vi "nonlinear spring simulation.vi"(7 "Solver Params":T1={"Initial Time"=0.0, "Final Time"=10.0, "Time Step"=0.1, "Absolute Tolerance"=0.001, "Relative Tolerance"=1e-07, "Solver Method"=enum."Runge-Kutta 4", "Discrete Time Step"=0.1, "Minimum Time Step"=0.01, "Maximum Time Step"=0.1, "Initial Time Step"=0.01} {"Initial Time Step" min=0.0; "Maximum Time Step" min=0.0; "Minimum Time Step" min=0.0; "Discrete Time Step" min=0.0; "Relative Tolerance" min=0.0; "Absolute Tolerance" min=0.0; "Time Step" min=0.0}, 8 "Error In":errorcluster, 9 "xp Noise STD":dbl(knob)=0.05 scale=0.0..0.1, 10 "Spring Constant":dbl(knob)=2.0 scale=0.0..10.0, 11 "Initial Conditions":dbl[](array[numeric])=[1.0, 0.0]) -> (0 "Error Out":errorcluster, 2 "times":dbl[](array[numeric]), 3 "outputs":dbl[][](array[numeric]))   [LabVIEW 2023]
doc: "Nonlinear spring simulation"
uses:
  <vilib>/gmath/NI_Gmath.lvlib
  <vilib>/Analysis/NI_AALBase.lvlib
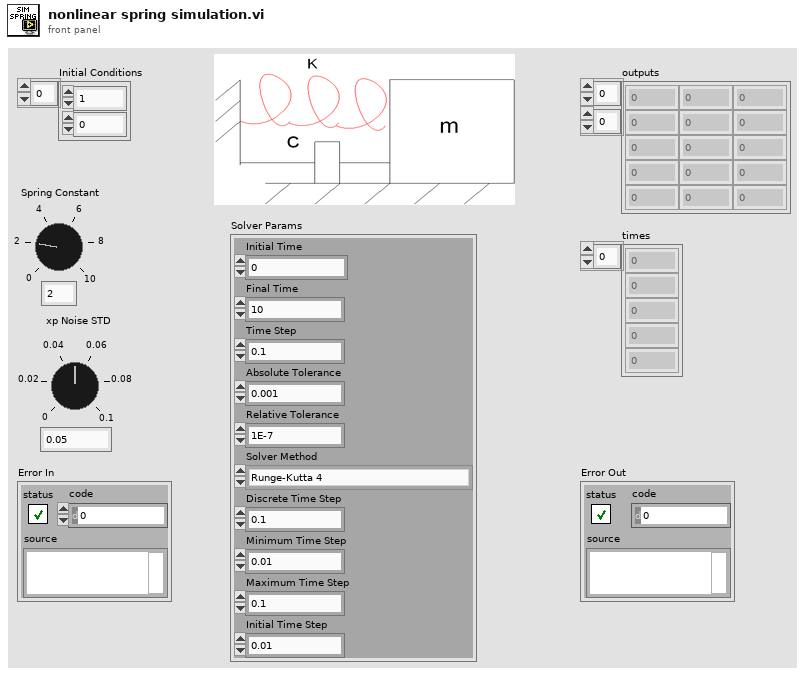
[diagram p1: front panel]
types:
  T1 = cluster{"Initial Time":dbl, "Final Time":dbl, "Time Step":dbl, "Absolute Tolerance":dbl, "Relative Tolerance":dbl, "Solver Method":enum16{"Runge-Kutta 1 (Euler)", "Runge-Kutta 2", "Runge-Kutta 3", "Runge-Kutta 4", "Runge-Kutta 23 (variable)", "Runge-Kutta 45 (variable)", "BDF (variable)", "Adams-Moulton (variable)", "Rosenbrock (variable)", "Discrete States Only"}, "Discrete Time Step":dbl, "Minimum Time Step":dbl, "Maximum Time Step":dbl, "Initial Time Step":dbl}
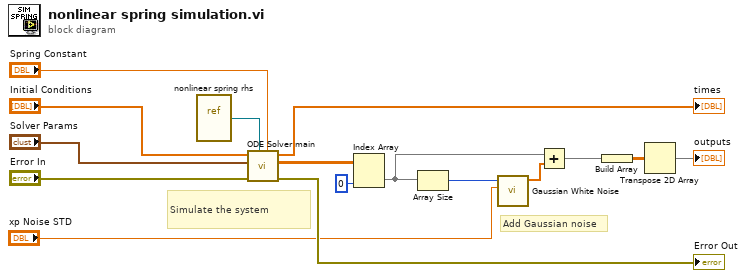
[diagram p0: block diagram]
diagram:
  # "Add Gaussian noise"
  # "Simulate the system"
  n1 = vi-ref "nonlinear spring rhs.vi"() -> (w11:refnum<vi>)
  n2 = call <vilib>:"ODE Solver main.vi"("data"="Spring Constant", "ODE F(X,t)"=w11, "error in (no error)"="Error In", "simulation parameters"="Solver Params", "x0"="Initial Conditions") -> ("error out"=→"Error Out":errorcluster, "outputs"=w12:dbl[][], "times"=→"times":dbl[])  [unwired: 4 in]
  n3 = Index Array(array=w12, index (col)=0 ("index (row)")) -> (element=w3:dbl[])  [unwired: 1 in]
  n4 = Array Size(array=w3) -> (size(s)=w15:i32)
  n5 = call <vilib>:"Gaussian White Noise.vi"("standard deviation"="xp Noise STD", "samples"=w15) -> ("Gaussian noise pattern"=w14:dbl[])  [unwired: 8 in, 1 out]
  n6 = Add(x=w3, y=w14) -> (x+y=w4:dbl[])
  n7 = Build Array(w4) -> (w16:dbl[][])
  n8 = Transpose 2D Array(2D array=w16) -> (transposed array=→"outputs":dbl[][])
